vi "fuzzy test.vi"() -> ()   [LabVIEW 2015]
uses:
  <vilib>/addons/Fuzzy Logic/FL Fuzzy Controller (SISO).vi
  <vilib>/addons/Fuzzy Logic/NI_Fuzzy_Logic_API.lvlib
panel:
  out "error out":errorcluster
  out "XY Graph":cluster{dbl[], dbl[]}(graph)
  in  "value":bool
  in  "y":dbl
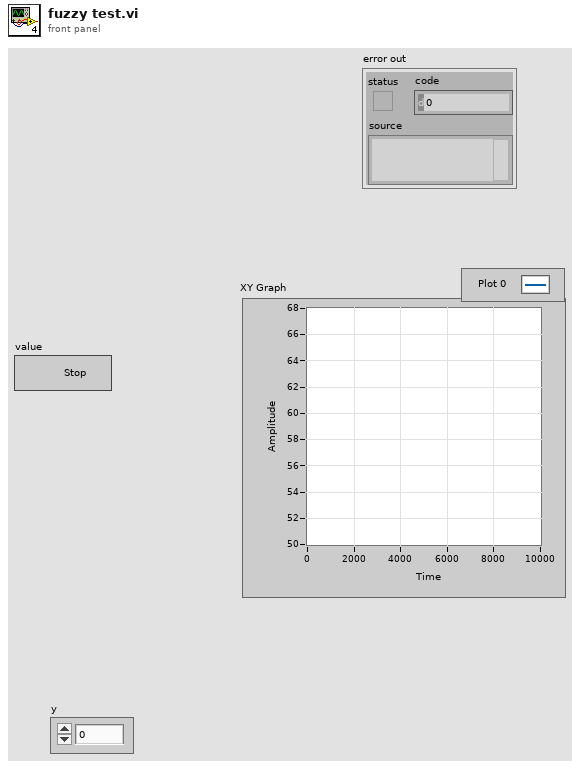
[diagram p1: front panel]
types:
  T1 = typedef "NI_Fuzzy_Logic_API.lvlib/FL System.ctl" = cluster{"input variables":T2[], "output variables":T2[], "rules":T5[], "defuzzification method":T11, "description":string, "user MF interpolating polynomials":T12[]}
  T2 = typedef "NI_Fuzzy_Logic_API.lvlib/FL Variable.ctl" = cluster{"name":string, "range":dbl[], "MFs":T3[]}
  T3 = typedef "NI_Fuzzy_Logic_API.lvlib/FL Membership Function.ctl" = cluster{"name":string, "shape":T4, "points":dbl[], "color":u32, "user-defined shape index":i32}
  T4 = typedef "NI_Fuzzy_Logic_API.lvlib/FL Membership Function Shape.ctl" = u16
  T5 = typedef "NI_Fuzzy_Logic_API.lvlib/FL Rule.ctl" = cluster{"antecedents":T6[], "antecedent connective":T8, "consequents":T9[], "consequent implication":T10, "degree of support":dbl}
  T6 = typedef "NI_Fuzzy_Logic_API.lvlib/FL Antecedent.ctl" = cluster{"Var Index":i32, "MF Index":i32, "Cond":T7}
  T7 = typedef "NI_Fuzzy_Logic_API.lvlib/FL Modifier.ctl" = u16
  T8 = typedef "NI_Fuzzy_Logic_API.lvlib/FL Antecedent Connective.ctl" = u16
  T9 = typedef "NI_Fuzzy_Logic_API.lvlib/FL Consequent.ctl" = cluster{"Var Index":i32, "MF Index":i32, "Cond":T7}
  T10 = typedef "NI_Fuzzy_Logic_API.lvlib/FL Consequent Implication.ctl" = u16
  T11 = typedef "NI_Fuzzy_Logic_API.lvlib/FL Defuzzification.ctl" = u16
  T12 = typedef "NI_Fuzzy_Logic_API.lvlib/FL Interpolating polynomials.ctl" = cluster{"X":dbl[], "Y":dbl[], "Y(x) coeff":dbl[][], "X(y) coeff":dbl[][], "Area(y) coeff":dbl[][], "coa_x(y) coeff":dbl[][]}
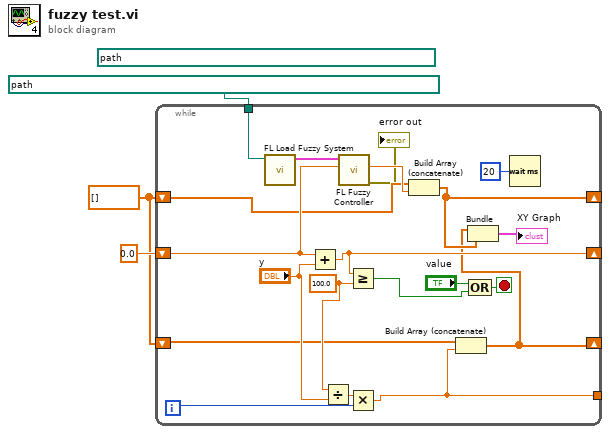
[diagram p0: block diagram]
diagram:
  (unwired) path "C:/Users/user/Desktop/0.0labview 電腦程式專用/growttt.fs" ("file path")
  w2 = dbl[] []
  n1 = while {
    tunnel: path "C:/Users/user/Desktop/0.0labview 電腦程式專用/growh curve ex function.fs" ("file path") -> [w22]
    shift-right: [w18] -> _
    shift-left: 0.0 -> [w21]
    shift-right: [w5] -> _
    shift-left: w2 -> [w12]
    tunnel: [w10] -> _
    shift-right: [w4] -> _
    shift-left: w2 -> [w11]
    i -> [w13]
    stop <- w19 stop-if-true
    w16 = 100.0 ("y")
    n2 = call <vilib>:"FL Load Fuzzy System.vi"("file path"=w22) -> ("fuzzy system out"=w23:T1)  [unwired: 9 in, 1 out]
    n3 = Add(x=w21, y="y") -> (x+y=w18:dbl)
    n4 = Divide(x=w16, y="y") -> (x/y=w14:dbl)
    n5 = call-poly <vilib>:"FL Fuzzy Controller.vi"("input value"=w21, "fuzzy system in"=w23) -> ("error out"=→"error out":errorcluster, "output value"=w20:dbl)  [unwired: 5 in, 3 out]
    n6 = Greater Or Equal?(x=w18, y=w16) -> (x >= y?=w6:bool)
    n7 = Multiply(x=w14, y=w13) -> (x*y=w10:dbl)
    n8 = Build Array (concatenate)(w12, w20) -> (w5:dbl[])
    n9 = Build Array (concatenate)(w11, w10) -> (w4:dbl[])
    n10 = Bundle(w4, w5) -> (→"XY Graph":cluster{dbl[], dbl[]})  [unwired: 1 in]
    n11 = Compound Arithmetic op=OR("value", w6) -> (w19:bool)
    n12 = Wait (ms)(milliseconds to wait=u32 20) -> ()  [unwired: 1 out]
  }
